vi "MW_Display_Py_Close_Device.vi"(0 "session in":refnum<k35>, 5 "module path":path=path "D:/dev/Guy_Storage/Work/Cancun/MW_Display_Test/Magewell Capture/Capture_LV.py", 11 "error in":errorcluster) -> (4 "session out":refnum<k35>, 6 "module path out":path, 14 "Close_Completed":bool, 15 "error out":errorcluster)   [LabVIEW 2023]
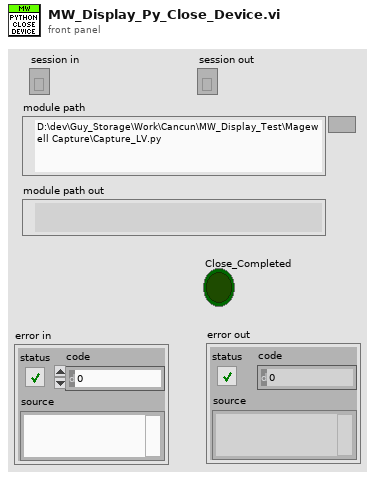
[diagram p1: front panel]
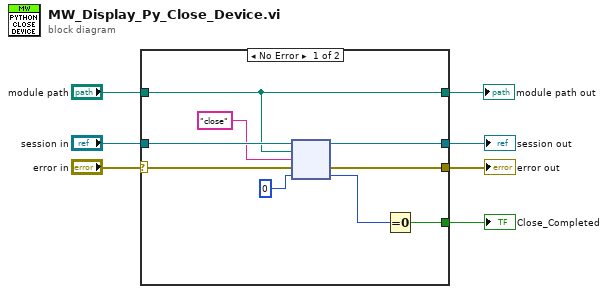
[diagram p0: block diagram]
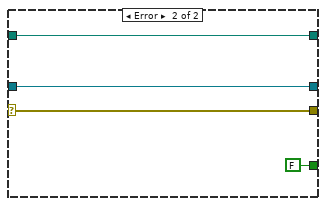
[diagram p2: hidden frame]
diagram:
  n1 = case shown="No Error" "error in" {
    selector: "error in" -> [w10 w19]
    tunnel: "module path" -> [w8 w17]
    tunnel: "session in" -> [w15 w20]
    tunnel: [w13 FALSE] -> w5
    tunnel: [w12 w19] -> w2
    tunnel: [w11 w20] -> w4
    tunnel: [w8 w17] -> w1
    frame No Error {
      n2 = node(w15, w8, "close" ("function name"), w10, 0) -> (w11:refnum<k35>, w12:errorcluster, w14:i32)  [unwired: 2 out]
      n3 = Equal To 0?(x=w14) -> (x = 0?=w13:bool)
    }
    frame Error {
    }
  }
  "Close_Completed" <- w5
  "session out" <- w4
  "error out" <- w2
  "module path out" <- w1
